vi "Electronic Procedure Debug.vi"() -> ()   [LabVIEW 2017]
panel:
  in  "CTAH outlet temperature":dbl
  in  "mass flow rate":dbl
  in  "NG flow rate":dbl
  in  "shaft RPM":dbl
  in  "NG pressure in":dbl
  in  "NG temperature in":dbl
  in  "LPT pressure ratio":dbl
  in  "HPT pressure ratio":dbl
  in  "CTAH frequency":dbl
  in  "desired power":dbl
  in  "pump frequency":dbl
  # "Do NOT run this during an experiment!"
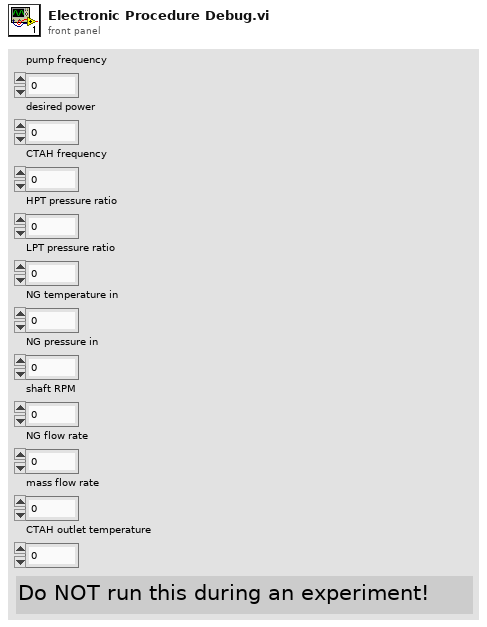
[diagram p1: front panel]
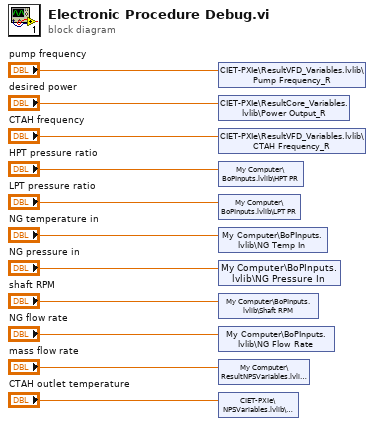
[diagram p0: block diagram]
diagram:
  n1 = shared-variable "CIET-PXIe\\ResultVFD_Variables.lvlib\\Pump Frequency_R"("pump frequency") -> ()  [unwired: 1 in, 1 out]
  n2 = shared-variable "CIET-PXIe\\ResultCore_Variables.lvlib\\Power Output_R"("desired power") -> ()  [unwired: 1 in, 1 out]
  n3 = shared-variable "CIET-PXIe\\ResultVFD_Variables.lvlib\\CTAH Frequency_R"("CTAH frequency") -> ()  [unwired: 1 in, 1 out]
  n4 = shared-variable "My Computer\\BoPInputs.lvlib\\HPT PR"("HPT pressure ratio") -> ()  [unwired: 1 in, 1 out]
  n5 = shared-variable "My Computer\\BoPInputs.lvlib\\LPT PR"("LPT pressure ratio") -> ()  [unwired: 1 in, 1 out]
  n6 = shared-variable "My Computer\\BoPInputs.lvlib\\NG Temp In"("NG temperature in") -> ()  [unwired: 1 in, 1 out]
  n7 = shared-variable "My Computer\\BoPInputs.lvlib\\NG Pressure In"("NG pressure in") -> ()  [unwired: 1 in, 1 out]
  n8 = shared-variable "My Computer\\BoPInputs.lvlib\\Shaft RPM"("shaft RPM") -> ()  [unwired: 1 in, 1 out]
  n9 = shared-variable "My Computer\\BoPInputs.lvlib\\NG Flow Rate"("NG flow rate") -> ()  [unwired: 1 in, 1 out]
  n10 = shared-variable "My Computer\\ResultNPSVariables.lvlib\\FM-40_R"("mass flow rate") -> ()  [unwired: 1 in, 1 out]
  n11 = shared-variable "CIET-PXIe\\NPSVariables.lvlib\\WT-40"("CTAH outlet temperature") -> ()  [unwired: 1 in, 1 out]
